vi "DualSVPWM_Timing_gen.vi"(0 "ref_beta":sgl[](array[numeric])=[0.0, 0.0], 5 "Period":i32=1, 7 "ref_max":sgl=0.9999695, 9 "input valid":bool=TRUE, 11 "ref_alpha":sgl[](array[numeric])=[0.0, 0.0]) -> (4 "C_timing":cluster{"ON":u32, "OFF":u32}[](array[cluster]), 6 "B_timing":cluster{"ON":u32, "OFF":u32}[](array[cluster]), 8 "A_timing":cluster{"ON":u32, "OFF":u32}[](array[cluster]), 10 "output valid":bool, 14 "feedback signals":cluster{"ready for input":bool})   [LabVIEW 2017]
doc: "This VI is created by the NI LabVIEW 2017 FPGA IP Builder.\n\nProject: SVPWM_dev.lvproj\nTarget: FPGA Target (sbRIO-9607)/IP Builder\nBuild Specification: Dual_SVPWM_TimingGen_SGL_gen\nDirectives Item: Dual_SVPWM_TimingGen_SGL_src\nTop-Level VI: C:\\PowerElectronicControl\\SpaceVectorPWM\\dev\\IPBuilder\\Dual_SVPWM_TimingGen_SGL_src.vi\n\nQuick Device Utilization Estimate\n--------------------------------------------\nSlice Registers: 2.4% (2503 out of 106400)\nSlice LUTs: 16.3% (8676 out of 53200)\nDSP48s: 4.1% (9 out of 220)\nBlock RAMs: 0.0% (0 out of 280)\n\nQuick Performance Estimate\n--------------------------------------------\nClock rate (MHz): 45.83\nInitiation interval (cycles): 40\nPipeline type: Not pipelined\nMinimum latency: 39\nMaximum latency: 39"
uses:
  <vilib>/rvi/IPIntegrationNode/IPINode_Typedef/niFpgaIPINodeSupportedFamilies.ctl
  <vilib>/rvi/IPIntegrationNode/IPINode_Utilities/niFpgaIPINodeSimCore.vi
  <vilib>/rvi/IPIntegrationNode/IPINode_Xnode/niFpgaIPINode.xnode
  DualSVPWM_Timing_gen Support/IPBlockSimFiles/xsim.dir/m99DA8A6E_topH/xsimkA98CB83324B04C5484BB4AC249155E1E.dll
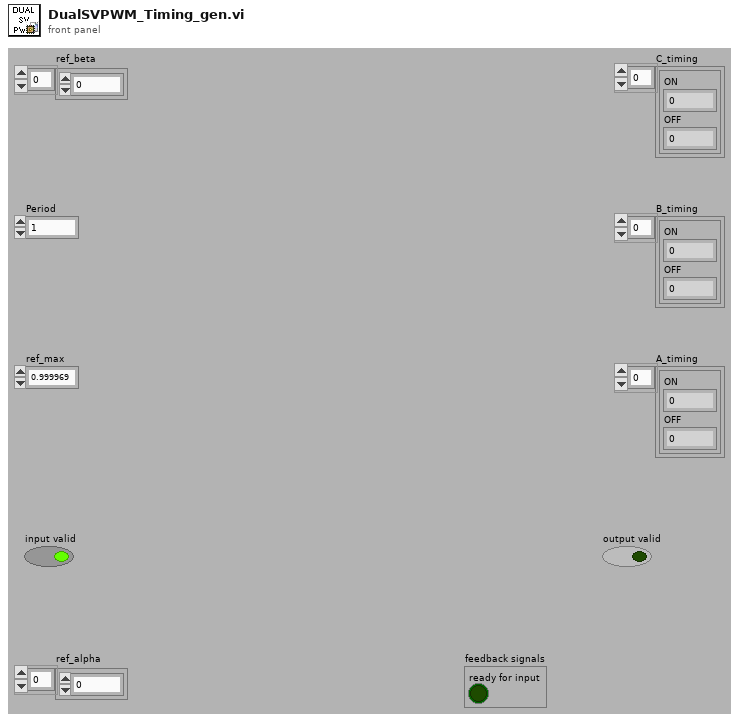
[diagram p1: front panel]
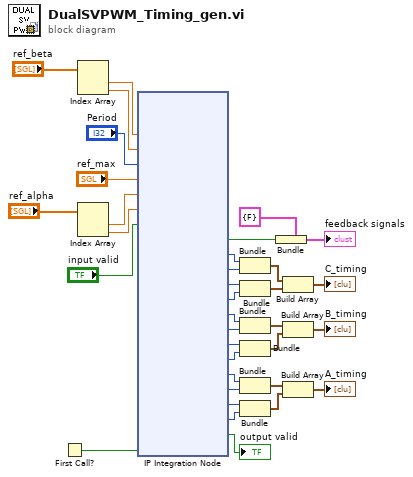
[diagram p0: block diagram]
diagram:
  n1 = First Call?() -> (First Call?: T/F=w35:bool)
  n2 = Index Array(array="ref_beta") -> (element #1=w17:sgl, element #2=w18:sgl)  [unwired: 2 in]
  n3 = Index Array(array="ref_alpha") -> (element #1=w13:sgl, element #2=w14:sgl)  [unwired: 2 in]
  n4 = xnode "IP Integration Node"("p_5_0"=w17, "p_5_1"=w18, "p_2"="Period", "p_1"="ref_max", "p_0_0"=w13, "p_0_1"=w14, "input_valid"="input valid", "first_call"=w35) -> ("ready_for_input"=w32:bool, "p_8_0_e_0"=w9:u32, "p_8_0_e_1"=w10:u32, "p_8_1_e_0"=w11:u32, "p_8_1_e_1"=w12:u32, "p_6_0_e_0"=w5:u32, "p_6_0_e_1"=w6:u32, "p_6_1_e_0"=w7:u32, "p_6_1_e_1"=w8:u32, "p_4_0_e_0"=w1:u32, "p_4_0_e_1"=w2:u32, "p_4_1_e_0"=w3:u32, "p_4_1_e_1"=w4:u32, "output_valid"=→"output valid":bool)  [unwired: 2 in]
  n5 = Bundle("p_8_0_e_0"=w9, "p_8_0_e_1"=w10) -> (w25:cluster{"p_8_0_e_0":u32, "p_8_0_e_1":u32})  [unwired: 1 in]
  n6 = Bundle("p_8_1_e_0"=w11, "p_8_1_e_1"=w12) -> (w26:cluster{"p_8_1_e_0":u32, "p_8_1_e_1":u32})  [unwired: 1 in]
  n7 = Bundle("p_6_0_e_0"=w5, "p_6_0_e_1"=w6) -> (w22:cluster{"p_6_0_e_0":u32, "p_6_0_e_1":u32})  [unwired: 1 in]
  n8 = Bundle("p_6_1_e_0"=w7, "p_6_1_e_1"=w8) -> (w23:cluster{"p_6_1_e_0":u32, "p_6_1_e_1":u32})  [unwired: 1 in]
  n9 = Bundle("p_4_0_e_0"=w1, "p_4_0_e_1"=w2) -> (w19:cluster{"p_4_0_e_0":u32, "p_4_0_e_1":u32})  [unwired: 1 in]
  n10 = Bundle("p_4_1_e_0"=w3, "p_4_1_e_1"=w4) -> (w20:cluster{"p_4_1_e_0":u32, "p_4_1_e_1":u32})  [unwired: 1 in]
  n11 = Bundle ("Bundle_feedback")(cluster=cluster{"ready for input":bool} {"ready for input"=FALSE}, "ready for input"=w32) -> (→"feedback signals":cluster{"ready for input":bool})
  n12 = Build Array(w25, w26) -> (→"C_timing":cluster{"p_8_1_e_0":u32, "p_8_1_e_1":u32}[])
  n13 = Build Array(w22, w23) -> (→"B_timing":cluster{"p_6_1_e_0":u32, "p_6_1_e_1":u32}[])
  n14 = Build Array(w19, w20) -> (→"A_timing":cluster{"p_4_1_e_0":u32, "p_4_1_e_1":u32}[])
